vi "convertpreampsens.vi"(2 "Preamp Sensitivity":T1(ring)=enum."100nA/V") -> (0 "Sensitivity":dbl)   [LabVIEW 2013]
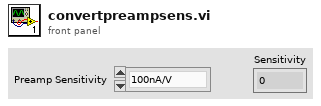
[diagram p1: front panel]
types:
  T1 = enum16{"1pA/V", "2pA/V", "5pA/V", "10pA/V", "20pA/V", "50pA/V", "100pA/V", "200pA/V", "500pA/V", "1nA/V", "2nA/V", "5nA/V", "10nA/V", "20nA/V", "50nA/V", "100nA/V", "200nA/V", "500nA/V", "1uA/V", "2uA/V", "5uA/V", "10uA/V", "20uA/V", "50uA/V", "100uA/V", "200uA/V", "500uA/V", "1mA/V"}
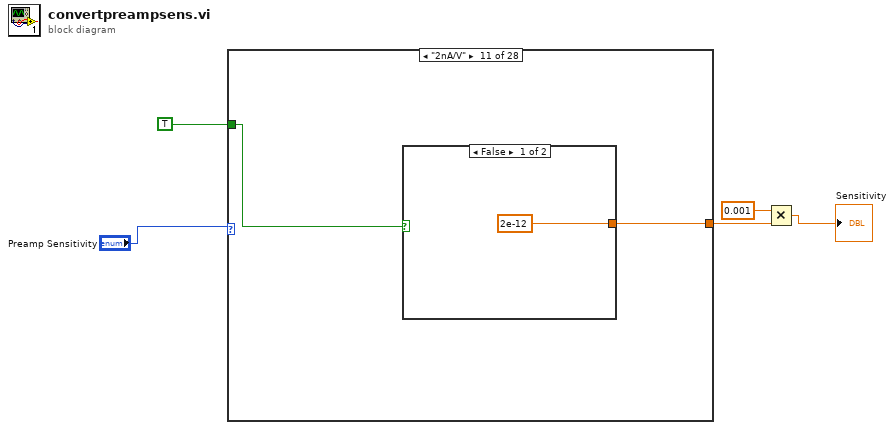
[diagram p0: block diagram]
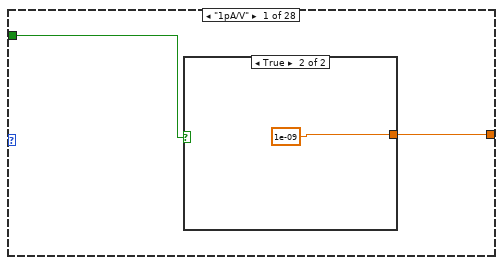
[diagram p2: hidden frame]
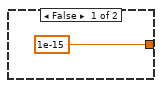
[diagram p3: hidden frame]
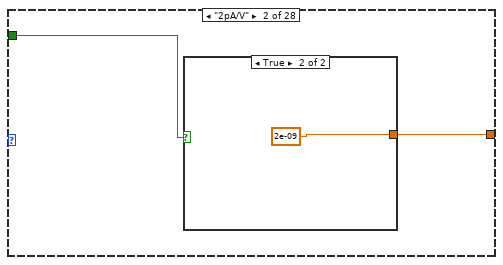
[diagram p4: hidden frame]
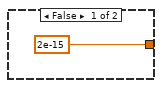
[diagram p5: hidden frame]
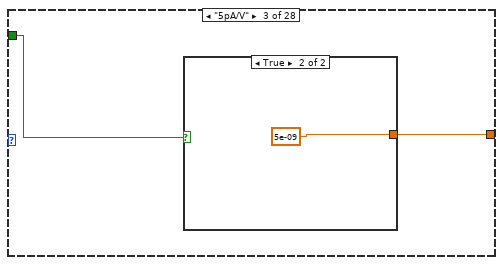
[diagram p6: hidden frame]
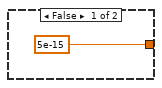
[diagram p7: hidden frame]
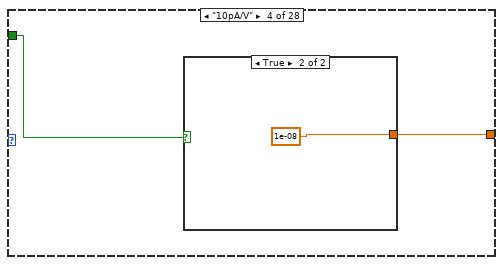
[diagram p8: hidden frame]
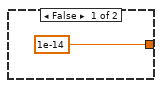
[diagram p9: hidden frame]
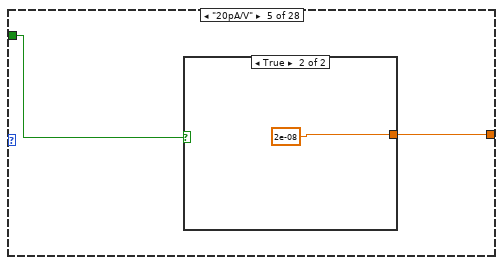
[diagram p10: hidden frame]
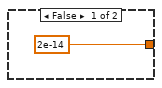
[diagram p11: hidden frame]
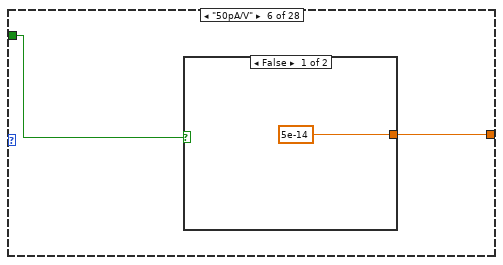
[diagram p12: hidden frame]
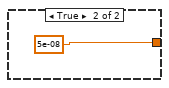
[diagram p13: hidden frame]
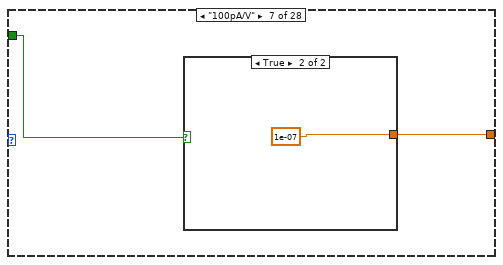
[diagram p14: hidden frame]
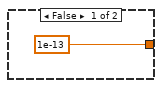
[diagram p15: hidden frame]
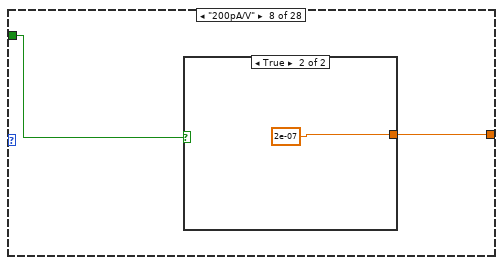
[diagram p16: hidden frame]
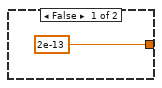
[diagram p17: hidden frame]
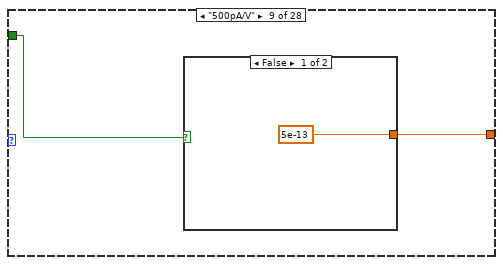
[diagram p18: hidden frame]
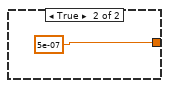
[diagram p19: hidden frame]
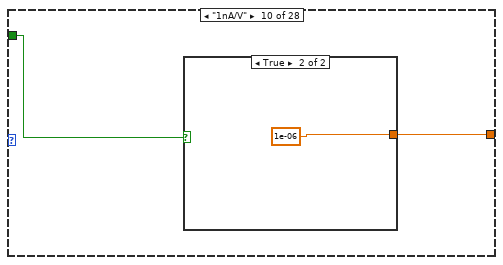
[diagram p20: hidden frame]
diagram:
  n1 = case shown="\"2nA/V\"" "Preamp Sensitivity" {
    tunnel: [w7 w11 w15 w19 w23 w27 w31 w35 w39 w43 w47 w51 w55 w59 w63 w67 w71 w75 w79 w83 w87 w91 w95 w99 w103 w107 w111 w115] -> w3
    tunnel: TRUE ("Voltage(T) Current(F)") -> [w6 w10 w14 w18 w22 w26 w30 w34 w38 w42 w46 w50 w54 w58 w62 w66 w70 w74 w78 w82 w86 w90 w94 w98 w102 w106 w110 w114]
    frame "1pA/V" {
      n2 = case shown="True" w6 {
        tunnel: [1e-15 1e-09] -> w7
        frame False {
        }
        frame True {
        }
      }
    }
    frame "2pA/V" {
      n3 = case shown="True" w10 {
        tunnel: [2e-15 2e-09] -> w11
        frame False {
        }
        frame True {
        }
      }
    }
    frame "5pA/V" {
      n4 = case shown="True" w14 {
        tunnel: [5e-15 5e-09] -> w15
        frame False {
        }
        frame True {
        }
      }
    }
    frame "10pA/V" {
      n5 = case shown="True" w18 {
        tunnel: [1e-14 1e-08] -> w19
        frame False {
        }
        frame True {
        }
      }
    }
    frame "20pA/V" {
      n6 = case shown="True" w22 {
        tunnel: [2e-14 2e-08] -> w23
        frame False {
        }
        frame True {
        }
      }
    }
    frame "50pA/V" {
      n7 = case shown="False" w26 {
        tunnel: [5e-14 5e-08] -> w27
        frame False {
        }
        frame True {
        }
      }
    }
    frame "100pA/V" {
      n8 = case shown="True" w30 {
        tunnel: [1e-13 1e-07] -> w31
        frame False {
        }
        frame True {
        }
      }
    }
    frame "200pA/V" {
      n9 = case shown="True" w34 {
        tunnel: [2e-13 2e-07] -> w35
        frame False {
        }
        frame True {
        }
      }
    }
    frame "500pA/V" {
      n10 = case shown="False" w38 {
        tunnel: [5e-13 5e-07] -> w39
        frame False {
        }
        frame True {
        }
      }
    }
    frame "1nA/V" {
      n11 = case shown="True" w42 {
        tunnel: [1e-12 1e-06] -> w43
        frame False {
        }
        frame True {
        }
      }
    }
    frame "2nA/V" {
      n12 = case shown="False" w46 {
        tunnel: [2e-12 2e-06] -> w47
        frame False {
        }
        frame True {
        }
      }
    }
    frame "5nA/V" {
      n13 = case shown="True" w50 {
        tunnel: [5e-12 5e-06] -> w51
        frame False {
        }
        frame True {
        }
      }
    }
    frame "10nA/V" {
      n14 = case shown="False" w54 {
        tunnel: [1e-11 1e-05] -> w55
        frame False {
        }
        frame True {
        }
      }
    }
    frame "20nA/V" {
      n15 = case shown="True" w58 {
        tunnel: [2e-11 2e-05] -> w59
        frame False {
        }
        frame True {
        }
      }
    }
    frame "50nA/V" {
      n16 = case shown="False" w62 {
        tunnel: [5e-11 5e-05] -> w63
        frame False {
        }
        frame True {
        }
      }
    }
    frame "100nA/V" {
      n17 = case shown="True" w66 {
        tunnel: [1e-10 0.0001] -> w67
        frame False {
        }
        frame True {
        }
      }
    }
    frame "200nA/V" {
      n18 = case shown="False" w70 {
        tunnel: [2e-10 0.0002] -> w71
        frame False {
        }
        frame True {
        }
      }
    }
    frame "500nA/V" {
      n19 = case shown="True" w74 {
        tunnel: [5e-10 0.0005] -> w75
        frame False {
        }
        frame True {
        }
      }
    }
    frame "1uA/V" {
      n20 = case shown="False" w78 {
        tunnel: [1e-09 0.001] -> w79
        frame False {
        }
        frame True {
        }
      }
    }
    frame "2uA/V" {
      n21 = case shown="True" w82 {
        tunnel: [2e-09 0.002] -> w83
        frame False {
        }
        frame True {
        }
      }
    }
    frame "5uA/V" {
      n22 = case shown="False" w86 {
        tunnel: [5e-09 0.005] -> w87
        frame False {
        }
        frame True {
        }
      }
    }
    frame "10uA/V" {
      n23 = case shown="True" w90 {
        tunnel: [1e-08 0.01] -> w91
        frame False {
        }
        frame True {
        }
      }
    }
    frame "20uA/V" {
      n24 = case shown="False" w94 {
        tunnel: [2e-08 0.02] -> w95
        frame False {
        }
        frame True {
        }
      }
    }
    frame "50uA/V" {
      n25 = case shown="True" w98 {
        tunnel: [5e-08 0.05] -> w99
        frame False {
        }
        frame True {
        }
      }
    }
    frame "100uA/V" {
      n26 = case shown="False" w102 {
        tunnel: [1e-07 0.1] -> w103
        frame False {
        }
        frame True {
        }
      }
    }
    frame "200uA/V" {
      n27 = case shown="True" w106 {
        tunnel: [2e-07 0.2] -> w107
        frame False {
        }
        frame True {
        }
      }
    }
    frame "500uA/V" {
      n28 = case shown="False" w110 {
        tunnel: [5e-07 0.5] -> w111
        frame False {
        }
        frame True {
        }
      }
    }
    frame "1mA/V" {
      n29 = case shown="True" w114 {
        tunnel: [1e-06 1.0] -> w115
        frame False {
        }
        frame True {
        }
      }
    }
  }
  n30 = Multiply(x=0.001, y=w3) -> (x*y=→"Sensitivity":dbl)
